vi "opencomm.vi"(0 "VISA resource name":refnum<visa-resource-name>="ASRL2::INSTR", 1 "Baud-rate (57600)":u32=57600) -> (2 "duplicate VISA resource name":refnum<visa-resource-name>, 3 "Error":bool)   [LabVIEW 2020]
uses:
  <vilib>/Instr/_visa.llb/VISA Configure Serial Port (Instr).vi
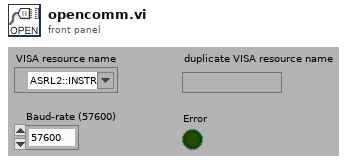
[diagram p1: front panel]
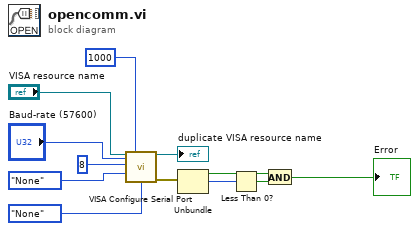
[diagram p0: block diagram]
diagram:
  n1 = call-poly "VISA Configure Serial Port"("VISA resource name"="VISA resource name", "timeout (10sec)"=u32 1000, "baud rate (9600)"="Baud-rate (57600)", "data bits (8)"=u16 8, "parity (0:none)"=enum16{"None", "Odd", "Even", "Mark", "Space"}."None", "flow control (0:none)"=enum16{"None", "XON/XOFF", "RTS/CTS"}."None" ("flow control (0:None)")) -> ("VISA resource name out"=→"duplicate VISA resource name":refnum<visa-resource-name>, "error out"=w6:errorcluster)  [unwired: 8 in]
  n2 = Unbundle(w6) -> ("status"=w3:bool, "code"=w5:i32)  [unwired: 1 out]
  n3 = Less Than 0?(x=w5) -> (x < 0?=w4:bool)
  n4 = And(x=w3, y=w4) -> (x .and. y?=→"Error":bool)
